vi "lua_gettable.vi"(8 "error in":errorcluster, 10 "int index":i32, 11 "lua_State *L":u64) -> (0 "error out":errorcluster)   [LabVIEW 2011]
doc: "void lua_gettable (lua_State *L, int index);\nPushes onto the stack the value t[k], where t is the value at the given valid index and k is the value at the top of the stack.\n\nThis function pops the key from the stack (putting the resulting value in its place). As in Lua, this function may trigger a metamethod for the \"index\" event (see §2.8)."
uses:
  lua5.1.dll
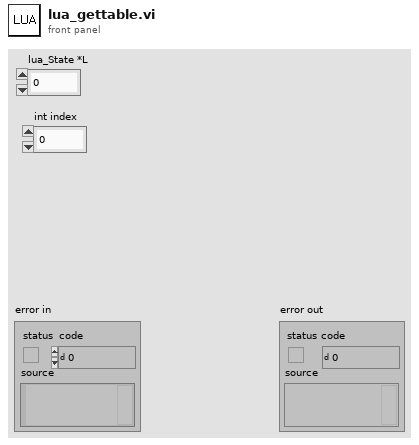
[diagram p1: front panel]
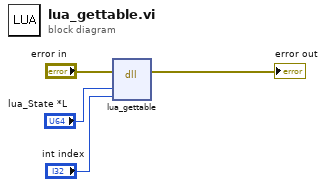
[diagram p0: block diagram]
diagram:
  n1 = dll-call lib="G:/_baidu_backup/monkey task 2012/source program/LuaDllToLabview/lowlevel/lua5.1.dll" fn="lua_gettable"(error in="error in", "lua_State *L"="lua_State *L", "int index"="int index") -> (error out=→"error out":errorcluster)  [unwired: 5 in, 1 out]
